vi "sr1.vi"() -> ()   [LabVIEW 2014]
panel:
  out "error out":errorcluster caption="错误输出"
  in  "重来":bool
  out "系统回应":string caption="标准输出"
  out "storelist":string[][](array[string])
  out "系统回应":string caption="标准输出"
  out "CM #":i32=-1
  out "系统回应":string caption="标准输出"
  out "系统回应":string caption="标准输出"
  out "显示窗口":string
  out "输入指令":string
  out "InstructionIn":string
  in  "停止":bool
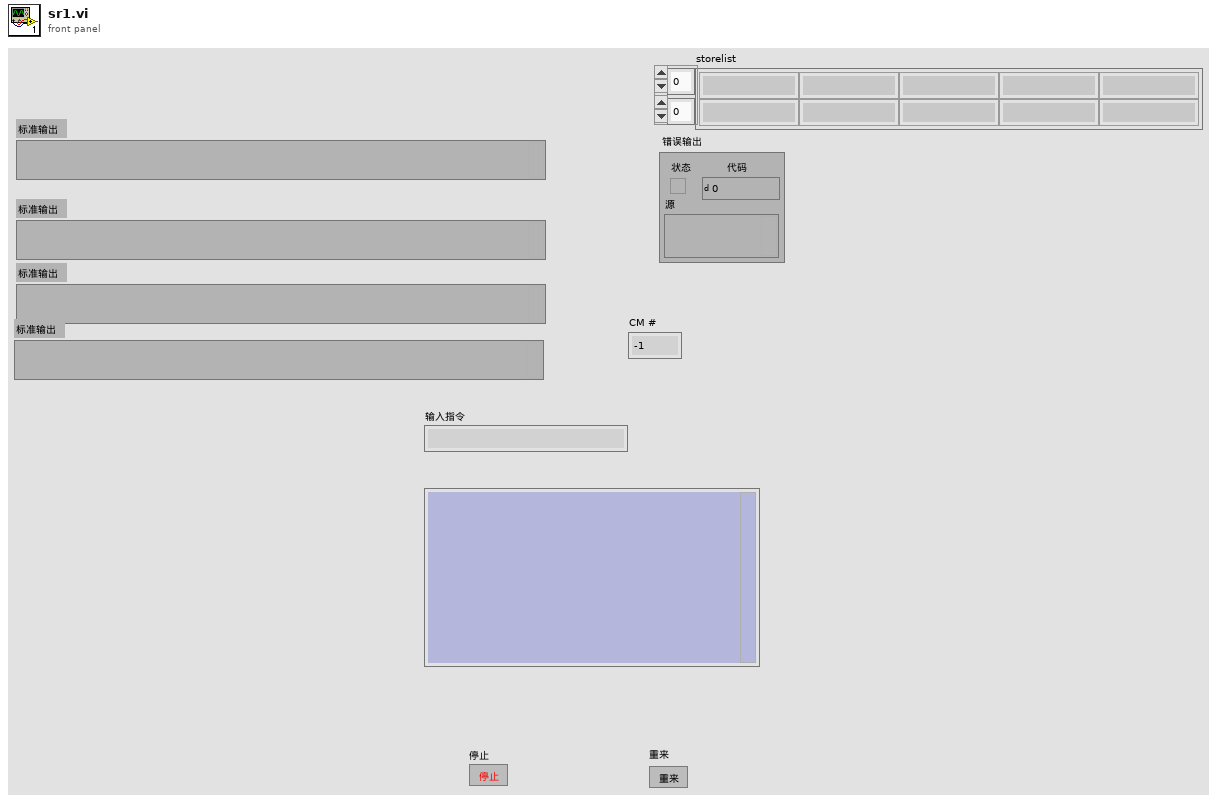
[diagram p1: front panel]
types:
  T1 = cluster{"输出数组":string[][], "CM #":i32, i32, string}
  T2 = enum16{"open", "replace", "create", "open or create", "replace or create", "replace or create with confirmation"}
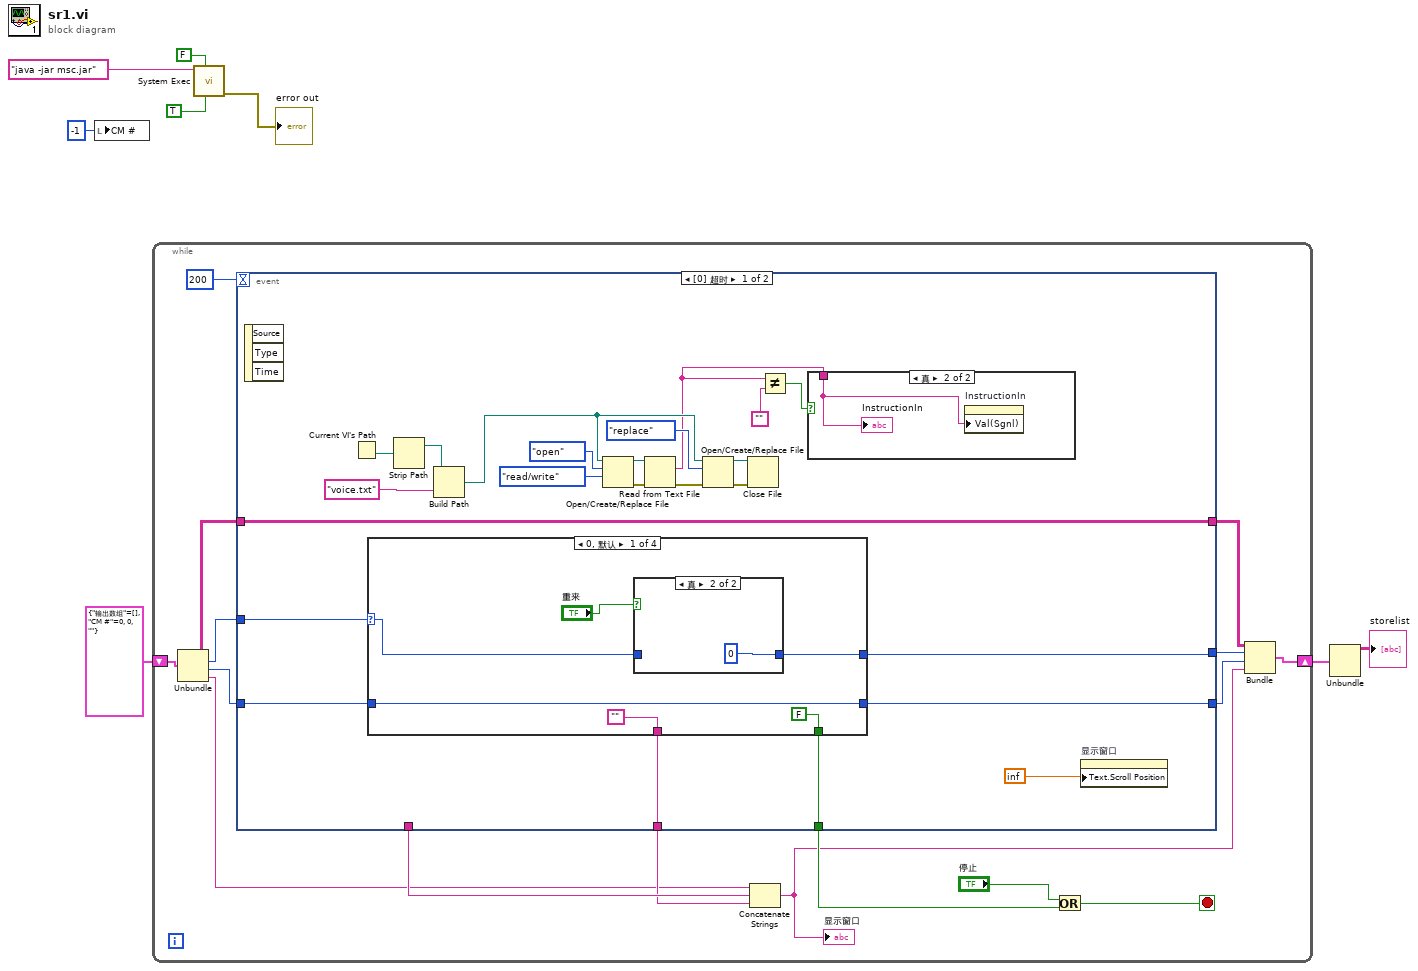
[diagram p0: block diagram]
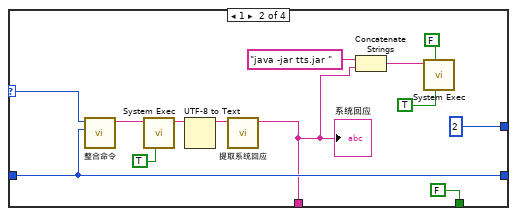
[diagram p3: hidden frame]
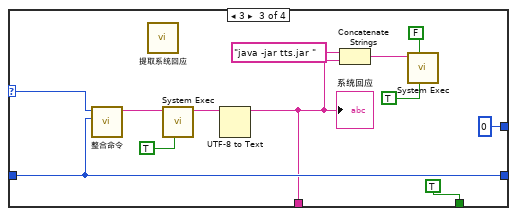
[diagram p4: hidden frame]
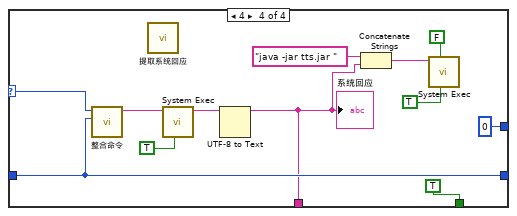
[diagram p5: hidden frame]
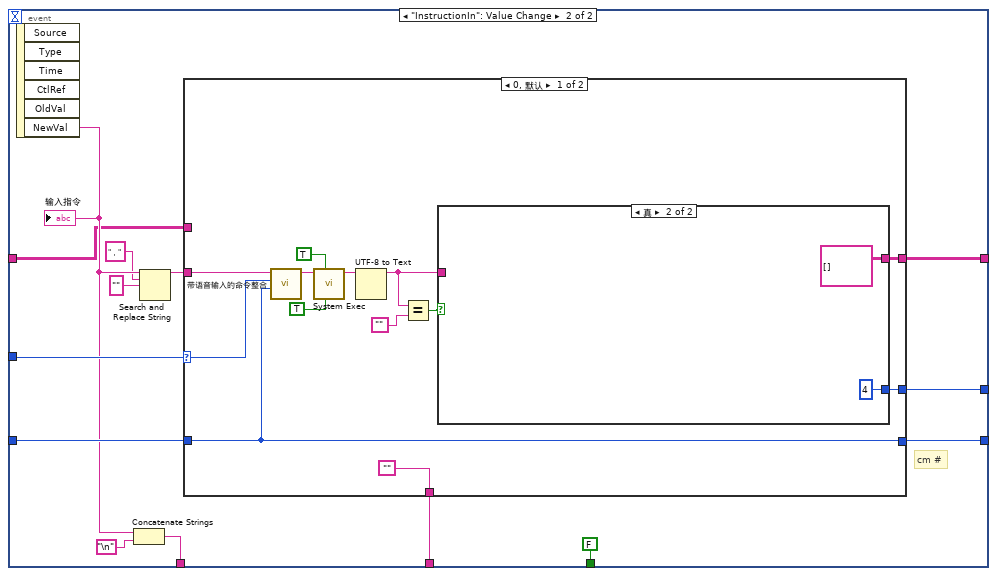
[diagram p7: hidden frame]
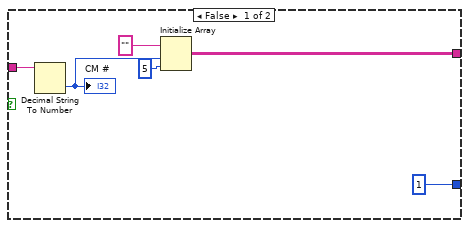
[diagram p8: hidden frame]
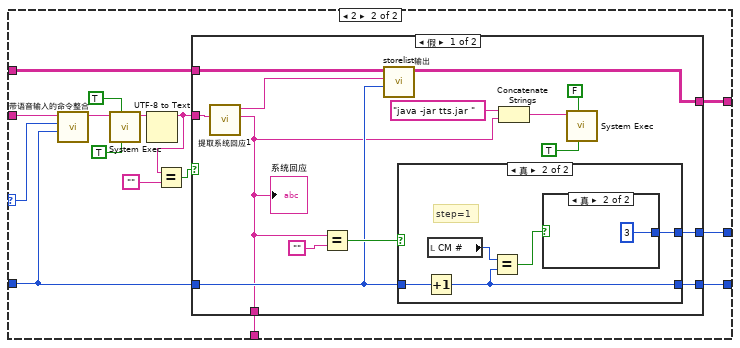
[diagram p9: hidden frame]
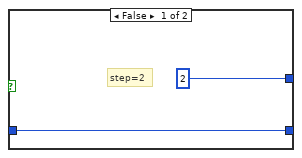
[diagram p10: hidden frame]
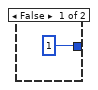
[diagram p11: hidden frame]
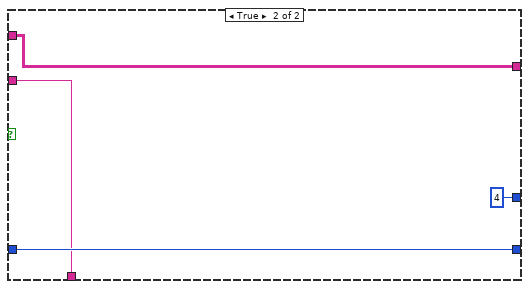
[diagram p12: hidden frame]
diagram:
  n1 = local write "CM #"(-1 ("CM #")) -> ()
  n2 = while {
    shift-right: [w13] -> w3
    shift-left: T1 {"输出数组"=[], "CM #"=0, 0, ""} -> [w18]
    stop <- w22 stop-if-true
    n3 = Unbundle(w18) -> ("输出数组"=w9:string[][], "CM #"=w10:i32, w11:i32, w12:string)
    n4 = event shown="[0] 超时" {
      selector: _ -> [_ _]
      dyn-events: _ -> [_ _]
      timeout: 200 -> [_ _]
      tunnel: w10 -> [w31 w107]
      tunnel: [w32 w104] -> w20
      tunnel: [w27 w106] -> w19
      tunnel: w11 -> [w28 w105]
      tunnel: [w30 FALSE] -> w21
      tunnel: [_ w101] -> w17
      tunnel: [w29 w103] -> w16
      tunnel: [w26 w95] -> w14
      tunnel: w9 -> [w26 w94]
      event Timeout {
        n5 = event-data() -> ()  [unwired: 1 in, 3 out]
        n6 = Current VI's Path() -> (path=w47:path)
        n7 = case shown="0, 默认" w31 {
          selector: w31 -> [w48 w63 w76 w88]
          tunnel: [w49 2 0 ("CM #") 0 ("CM #")] -> w32
          tunnel: w28 -> [w51 w61 w74 w86]
          tunnel: [FALSE FALSE TRUE TRUE] -> w30
          tunnel: ["" w56 w69 w81] -> w29
          tunnel: [w51 w61 w74 w86] -> w27
          frame 0, Default {
            n8 = case shown="真" "重来" {
              tunnel: [w54 0] -> w49
              tunnel: w48 -> [w54 _]
              frame False {
              }
              frame True {
              }
            }
          }
          frame 1 {
            n9 = call "整合命令.vi"("CM"=w61, "step"=w63) -> ("命令"=w62:string)  [unwired: 9 in]
            n10 = call <vilib>:"System Exec.vi"("run minimized? (F)"=TRUE, "command line"=w62) -> ("standard output"=w67:string)  [unwired: 6 in, 3 out]
            n11 = UTF-8 to Text(11:w67) -> (3:w66:string)  [unwired: 2 in, 1 out]
            n12 = call "提取系统回应.vi"("字符串"=w66) -> ("系统回应"=w56:string)  [unwired: 10 in]
            "系统回应" <- w56
            n13 = Concatenate Strings("java -jar tts.jar " ("command line"), w56) -> (w60:string)
            n14 = call <vilib>:"System Exec.vi"("run minimized? (F)"=TRUE, "wait until completion? (T)"=FALSE, "command line"=w60) -> ()  [unwired: 5 in, 4 out]
          }
          frame 3 {
            n15 = call "整合命令.vi"("CM"=w74, "step"=w76) -> ("命令"=w75:string)  [unwired: 9 in]
            n16 = call "提取系统回应.vi"() -> ()  [unwired: 11 in, 1 out]
            n17 = call <vilib>:"System Exec.vi"("run minimized? (F)"=TRUE, "command line"=w75) -> ("standard output"=w80:string)  [unwired: 6 in, 3 out]
            n18 = UTF-8 to Text(11:w80) -> (3:w69:string)  [unwired: 2 in, 1 out]
            "系统回应" <- w69
            n19 = Concatenate Strings("java -jar tts.jar " ("command line"), w69) -> (w73:string)
            n20 = call <vilib>:"System Exec.vi"("run minimized? (F)"=TRUE, "wait until completion? (T)"=FALSE, "command line"=w73) -> ()  [unwired: 5 in, 4 out]
          }
          frame 4 {
            n21 = call "整合命令.vi"("CM"=w86, "step"=w88) -> ("命令"=w87:string)  [unwired: 9 in]
            n22 = call "提取系统回应.vi"() -> ()  [unwired: 11 in, 1 out]
            n23 = call <vilib>:"System Exec.vi"("run minimized? (F)"=TRUE, "command line"=w87) -> ("standard output"=w92:string)  [unwired: 6 in, 3 out]
            n24 = UTF-8 to Text(11:w92) -> (3:w81:string)  [unwired: 2 in, 1 out]
            "系统回应" <- w81
            n25 = Concatenate Strings("java -jar tts.jar " ("command line"), w81) -> (w85:string)
            n26 = call <vilib>:"System Exec.vi"("run minimized? (F)"=TRUE, "wait until completion? (T)"=FALSE, "command line"=w85) -> ()  [unwired: 5 in, 4 out]
          }
        }
        n27 = Strip Path(path=w47) -> (stripped path=w44:path)  [unwired: 1 out]
        n28 = Build Path(base path=w44, name or relative path="voice.txt" ("名称或相对路径")) -> (appended path=w46:path)
        n29 = Open/Create/Replace File(file path (use dialog)=w46, operation (0:open)=T2."open" ("操作(0:open)"), access (0:read/write)=enum16{"read/write", "read-only", "write-only"}."read/write" ("权限(0:read/write)")) -> (refnum out=w39:refnum<file>, error out=w38:errorcluster)  [unwired: 3 in, 1 out]
        n30 = Read from Text File(file (use dialog)=w39, error in=w38) -> (text=w33:string, error out=w41:errorcluster)  [unwired: 2 in, 2 out]
        n31 = Open/Create/Replace File(file path (use dialog)=w46, error in=w41, operation (0:open)=T2."replace" ("操作(0:open)")) -> (refnum out=w42:refnum<file>, error out=w43:errorcluster)  [unwired: 3 in, 1 out]
        n32 = Close File(refnum=w42, error in=w43) -> ()  [unwired: 2 out]
        n33 = Not Equal?(x=w33, y="") -> (x != y?=w34:bool)
        n34 = case shown="真" w34 {
          tunnel: w33 -> [_ w93]
          frame False {
          }
          frame True {
            n35 = property on="InstructionIn" class="Str"("Val(Sgnl)"=w93) -> ()  [unwired: 2 in, 2 out]
            "InstructionIn" <- w93
          }
        }
        n36 = property on="显示窗口" class="Str"("Text.Scroll Position"=inf) -> ()  [unwired: 2 in, 2 out]
      }
      event "InstructionIn": Value Change {
        # "cm #"
        n37 = event-data() -> ("NewVal"=w100:string)  [unwired: 1 in, 5 out]
        "输入指令" <- w100
        n38 = Concatenate Strings(w100, "\n") -> (w101:string)
        n39 = Search and Replace String(input string=w100, search string="，" ("子字符串(\"\")"), replace string="" ("替换字符串(\"\")")) -> (result string=w97:string)  [unwired: 5 in, 3 out]
        n40 = case shown="0, 默认" w107 {
          selector: w107 -> [w115 w137]
          tunnel: [w114 w141] -> w106
          tunnel: w105 -> [w114 w134]
          tunnel: [w118 w140] -> w104
          tunnel: ["" w135] -> w103
          tunnel: w97 -> [w113 w138]
          tunnel: [w111 w132] -> w95
          tunnel: w94 -> [_ w133]
          frame 0, Default {
            n41 = call "带语音输入的命令整合.vi"("CM"=w114, "step"=w115, "输入指令"=w113) -> ("命令"=w112:string)  [unwired: 8 in]
            n42 = call <vilib>:"System Exec.vi"("run minimized? (F)"=TRUE, "wait until completion? (T)"=TRUE, "command line"=w112) -> ("standard output"=w119:string)  [unwired: 5 in, 3 out]
            n43 = UTF-8 to Text(11:w119) -> (3:w109:string)  [unwired: 2 in, 1 out]
            n44 = Equal?(x=w109, y="") -> (x = y?=w108:bool)
            n45 = case shown="真" w108 {
              tunnel: [1 4] -> w118
              tunnel: w109 -> [w125 _]
              tunnel: [w121 string[][] []] -> w111
              frame False {
                n46 = Decimal String To Number(string=w125) -> (number=w123:i32)  [unwired: 2 in, 1 out]
                "CM #" <- w123
                n47 = Initialize Array("", w123, 5 ("维数大小")) -> (w121:string[][])
              }
              frame True {
              }
            }
          }
          frame 2 {
            n48 = call "带语音输入的命令整合.vi"("CM"=w134, "step"=w137, "输入指令"=w138) -> ("命令"=w136:string)  [unwired: 8 in]
            n49 = call <vilib>:"System Exec.vi"("run minimized? (F)"=TRUE, "wait until completion? (T)"=TRUE, "command line"=w136) -> ("standard output"=w142:string)  [unwired: 5 in, 3 out]
            n50 = UTF-8 to Text(11:w142) -> (3:w130:string)  [unwired: 2 in, 1 out]
            n51 = Equal?(x=w130, y="") -> (x = y?=w129:bool)
            n52 = case shown="假" w129 {
              tunnel: [w155 w170] -> w141
              tunnel: [w154 4] -> w140
              tunnel: w130 -> [w153 w167]
              tunnel: [w144 w167] -> w135
              tunnel: w134 -> [w151 w170]
              tunnel: w133 -> [w150 w168]
              tunnel: [w149 w168] -> w132
              frame False {
                n53 = call "提取系统回应1.vi"("字符串"=w153) -> ("系统回应"=w144:string, "子字符串之前"=w152:string)  [unwired: 9 in]
                "系统回应" <- w144
                n54 = Equal?(x=w144, y="") -> (x = y?=w156:bool)
                n55 = call "storelist输出.vi"("CM"=w151, 10:"storelist"=w152, 11:"storelist"=w150) -> ("输出数组"=w149:string[][])  [unwired: 8 in]
                n56 = case shown="真" w156 {
                  tunnel: [2 w163] -> w154
                  tunnel: w151 -> [w159 w164]
                  tunnel: [w159 w160] -> w155
                  frame False {
                    # "step=2"
                  }
                  frame True {
                    # "step=1"
                    n57 = Increment(x=w164) -> (x+1=w160:i32)
                    n58 = local read "CM #"() -> (w162:i32)
                    n59 = Equal?(x=w162, y=w160) -> (x = y?=w161:bool)
                    n60 = case shown="真" w161 {
                      tunnel: [1 3] -> w163
                      frame False {
                      }
                      frame True {
                      }
                    }
                  }
                }
                n61 = Concatenate Strings("java -jar tts.jar " ("command line"), w144) -> (w148:string)
                n62 = call <vilib>:"System Exec.vi"("run minimized? (F)"=TRUE, "wait until completion? (T)"=FALSE, "command line"=w148) -> ()  [unwired: 5 in, 4 out]
              }
              frame True {
              }
            }
          }
        }
      }
    }
    n63 = Concatenate Strings(w12, w17, w16) -> (w15:string)
    "显示窗口" <- w15
    n64 = Or(x="停止", y=w21) -> (x .or. y?=w22:bool)
    n65 = Bundle("输出数组"=w14, "CM #"=w20, w19, w15) -> (w13:T1)  [unwired: 1 in]
  }
  n66 = call <vilib>:"System Exec.vi"("run minimized? (F)"=TRUE, "wait until completion? (T)"=FALSE, "command line"="java -jar msc.jar") -> ("error out"=→"error out":errorcluster)  [unwired: 5 in, 3 out]
  n67 = Unbundle(w3) -> ("输出数组"=→"storelist":string[][])  [unwired: 3 out]
